vi "Determine Winning Team.vi"(10 "Scores":i32[](array[numeric])=[3000, 0, 5000, 100]) -> (2 "Tie?":bool, 3 "Index of Winner":i32)   [LabVIEW 2023]
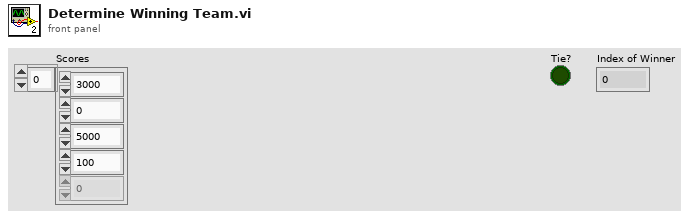
[diagram p1: front panel]
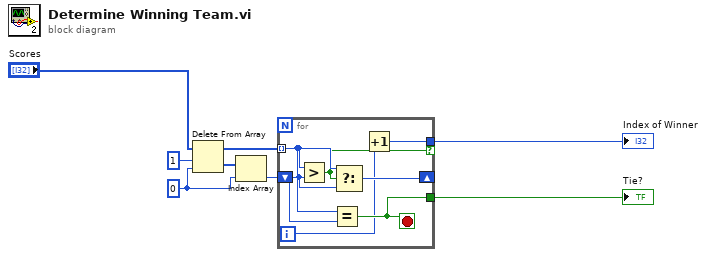
[diagram p0: block diagram]
diagram:
  w6 = 0 ("index")
  n1 = Delete From Array(array="Scores", length=1, index=w6) -> (deleted portion=w5:i32[], array with subset deleted=w7:i32[])
  n2 = Index Array(array=w5, index=w6) -> (element=w4:i32)
  n3 = for {
    shift-right: [w15] -> _
    shift-left: w4 -> [w13]
    tunnel: w7 -> [w14] mode=indexing
    tunnel: [w12] -> w2
    tunnel: [w10] -> w1 if=w9
    i -> [w11]
    stop <- w12 stop-if-true
    n4 = Greater?(x=w14, y=w13) -> (0:w9:bool)
    n5 = Equal?(x=w14, y=w13) -> (x = y?=w12:bool)
    n6 = Select(t=w14, s=w9, f=w13) -> (s? t:f=w15:i32)
    n7 = Increment(x=w11) -> (x+1=w10:i32)
  }
  "Tie?" <- w2
  "Index of Winner" <- w1
